vi "PCTx with dll.vi"() -> ()   [LabVIEW 2012]
uses:
  PCTx/PCTx.lvlib
panel:
  in  "Stop PCTx":bool
  in  "stop":bool
  out "Data Sent?":bool
  out "Connected?":bool
  in  "delay10":i32(slide)=512 min=0 max=1023 scale=0.0..3.0
  in  "delay8":i32(slide)=512 min=0 max=1023 scale=0.0..3.0
  in  "delay9":i32(slide)=512 min=0 max=1023 scale=0.0..255.0
  in  "delay7":i32(slide)=512 min=0 max=1023 scale=0.0..255.0
  in  "delay6":i32(slide)=512 min=0 max=1023 scale=0.0..3.0
  in  "delay5":i32(slide)=512 min=0 max=1023 scale=0.0..255.0
  in  "delay4":i32(slide)=512 min=0 max=1023 scale=0.0..3.0
  in  "delay3":i32(slide)=3 min=0 max=255 scale=0.0..255.0
  in  "delay2":i32(slide)=512 min=0 max=1023 scale=0.0..3.0
  in  "delay1":i32(slide) min=0 max=1023 scale=0.0..1023.0
  out "error out":errorcluster
  in  "error in":errorcluster
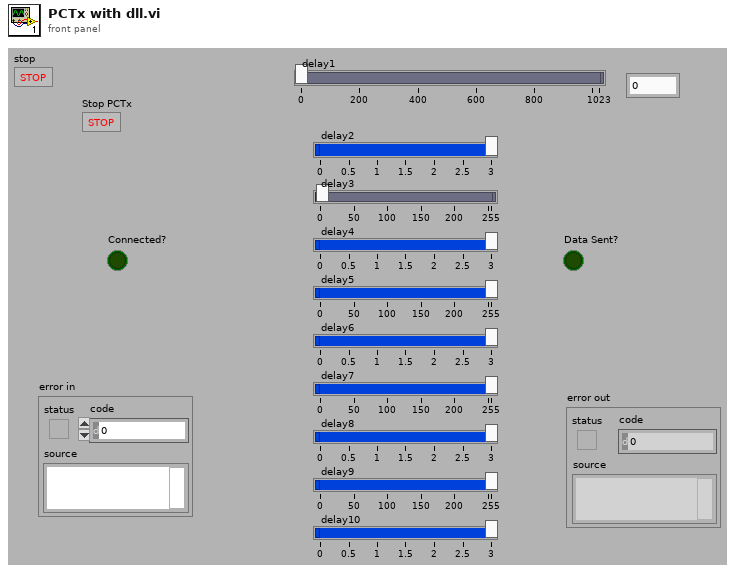
[diagram p1: front panel]
types:
  T1 = typedef "IMAQ Image.ctl" = refnum<image>
  T2 = typedef "IMAQ USB.ctl" = refnum<k1>
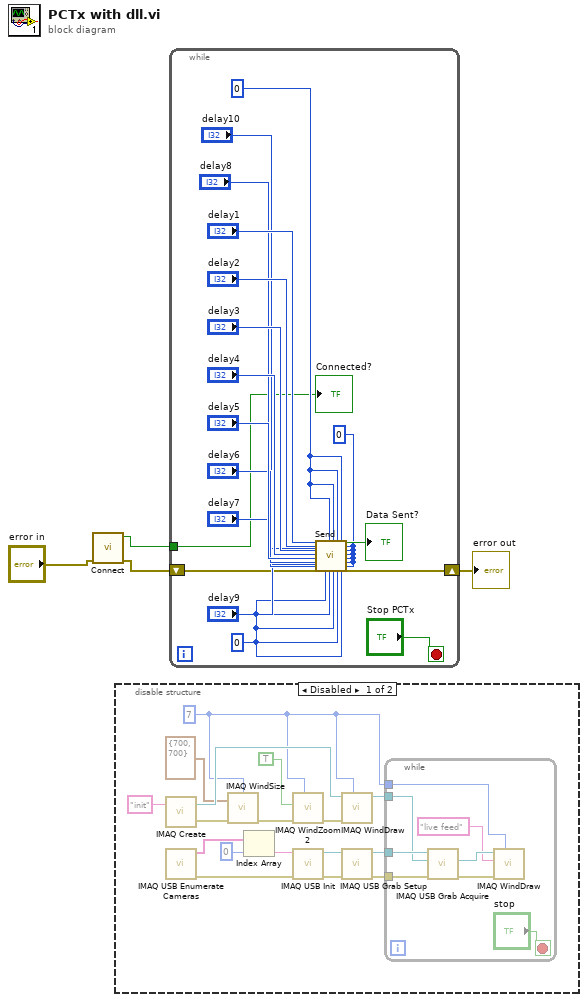
[diagram p0: block diagram]
diagram:
  n1 = call "Connect.vi"("error in (no error)"="error in") -> ("error out"=w2:errorcluster, "function return"=w1:bool)  [unwired: 9 in]
  n2 = disable-structure shown="Disabled" {
    frame Disabled {
      w5 = 7 ("Window Number (0...15)")
      n3 = call "IMAQ Create"("Image Name"="init") -> ("New Image"=w13:T1, "error out"=w12:errorcluster)  [unwired: 4 in]
      n4 = call <vilib>:"IMAQ USB Enumerate Cameras.vi"() -> ("error out"=w17:errorcluster, "USB Camera Names"=w16:string[])  [unwired: 10 in]
      n5 = call "IMAQ WindSize"("error in (no error)"=w12, "Width & Height"=cluster{"Width":i32, "Height":i32} {"Width"=700, "Height"=700}, "Window Number"=w5) -> ("error out"=w10:errorcluster)  [unwired: 3 in, 2 out]
      n6 = Index Array(array=w16, index=0) -> (element=w14:string)
      n7 = call "IMAQ WindZoom 2"("Window Number (0...15)"=w5, "error in (no error)"=w10, "Zoom to Fit? (False)"=TRUE) -> ("error out"=w8:errorcluster)  [unwired: 5 in, 3 out]
      n8 = call <vilib>:"IMAQ USB Init.vi"("error in (no error)"=w17, "USB Camera Name"=w14) -> ("error out"=w18:errorcluster, "IMAQ USB Session Out"=w19:T2)  [unwired: 8 in]
      n9 = call "IMAQ WindDraw"("Window Number (0...15)"=w5, "error in (no error)"=w8, "Image"=w13) -> ("Image Out (duplicate)"=w7:T1)  [unwired: 7 in, 1 out]
      n10 = call <vilib>:"IMAQ USB Grab Setup.vi"("error in (no error)"=w18, "IMAQ USB Session In"=w19) -> ("error out"=w20:errorcluster, "IMAQ USB Session Out"=w21:T2)  [unwired: 8 in]
      n11 = while {
        tunnel: w21 -> [w29]
        tunnel: w20 -> [w28]
        tunnel: w7 -> [w26]
        tunnel: w5 -> [w23]
        stop <- "stop" stop-if-true
        n12 = call <vilib>:"IMAQ USB Grab Acquire.vi"("error in (no error)"=w28, "Image in"=w26, "IMAQ USB Session In"=w29) -> ("error out"=w25:errorcluster, "Image out"=w24:T1)  [unwired: 6 in, 1 out]
        n13 = call "IMAQ WindDraw"("Window Number (0...15)"=w23, "error in (no error)"=w25, "Title"="live feed", "Image"=w24) -> ()  [unwired: 6 in, 2 out]
      }
    }
    frame Enabled {
    }
  }
  n14 = while {
    shift-right: [w47] -> w4
    shift-left: w2 -> [w30]
    tunnel: w1 -> [w31]
    stop <- "Stop PCTx" stop-if-true
    w33 = 0 ("delay25")
    w35 = 0 ("delay11")
    w36 = 0 ("delay12")
    n15 = call "Send.vi"("Ch1"="delay1", "Ch2"="delay2", "Ch3"="delay3", "Ch4"="delay4", "Ch5"="delay5", 5:"delay6", 6:"delay7", "error in (no error)"=w30, 8:"delay8", 9:"delay9", 10:"delay10", 11:w35, 12:w36, 13:w35, 14:w36, 15:w35, 16:w36, 17:w35, 18:w36, 19:w35, 21:w33, 22:w33, 23:w33, 24:w33, 25:w33, 26:w33) -> ("function return"=→"Data Sent?":bool, "error out"=w47:errorcluster)
    "Connected?" <- w31
  }
  "error out" <- w4
